vi "NI6602.Initialize.vi"(0 "i ref in":refnum<vi>, 2 "Counter Array":tag[](array[tag]), 5 "error in (no error)":errorcluster) -> (14 "i ref out":refnum<vi>, 16 "Task Array":refnum<k21>[](array[refnum]), 19 "error out":errorcluster)   [LabVIEW 2014, in "NI6602.lvlib"]
doc: "Initializes the device.\n\nLicense Agreement for this software:\n\nCopyright (C)\nGesellschaft für Schwerionenforschung, GSI\nPlanckstr. 1\n64291 Darmstadt\nGermany\n\nContact: D.Beck@gsi.de \n\nThis program is free software; you can redistribute it and/or modify it under the terms of the \nGNU General Public License as published by the Free Software Foundation; either version 2 of \nthe license, or (at your option) any later version.\n\nThis program is distributed in the hope that it will be useful, but WITHOUT ANY WARRANTY; \nwithout even the implied warranty of MERCHANTABILITY or FITNESS FOR A PARTICULAR PURPOSE. See the GNU General License for more details (http://www.gnu.org).\n\nGesellschaft für Schwerionenforschung, GSI\nPlanckstr. 1, 64291 Darmstadt, Germany\nFor all questions and ideas contact: M.Richter@gsi.de, H.Brand@gsi.de or D.Beck@gsi.de.\nLast update: 16-JUN-2004"
uses:
  NI6602.lvlib
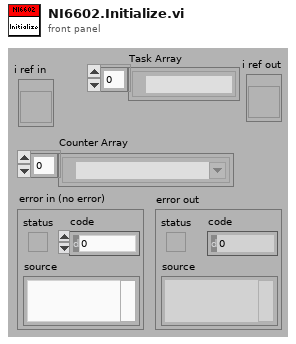
[diagram p1: front panel]
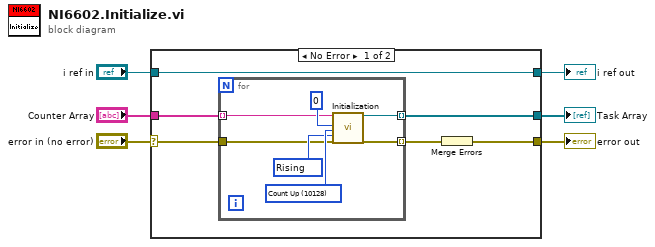
[diagram p0: block diagram]
diagram:
  n1 = case shown="No Error" "error in (no error)" {
    selector: "error in (no error)" -> [w9 w21]
    tunnel: [w10 w20] -> w6
    tunnel: [w11 w21] -> w5
    tunnel: "i ref in" -> [w10 w20]
    tunnel: "Counter Array" -> [w8 _]
    tunnel: [w7 _] -> w1
    frame No Error {
      n2 = for {
        tunnel: w9 -> [w16]
        tunnel: [w15] -> w12 mode=indexing
        tunnel: w8 -> [w14] mode=indexing
        tunnel: [w13] -> w7 mode=indexing
        w17 = 10280 items=["Rising"=10280, "Falling"=10171] ("edge")
        w18 = 10128 items=["Count Up"=10128, "Count Down"=10124, "Externally Controlled"=10326] ("count direction")
        n3 = call "Initialization.vi"("counter"=w14, "initial count"=u32 0, "count direction"=w18, "edge"=w17, "error in"=w16) -> ("task out"=w13:refnum<k21>, "error out"=w15:errorcluster)  [unwired: 13 in]
      }
      n4 = Merge Errors(w12) -> (w11:errorcluster)
    }
    frame Error {
    }
  }
  "i ref out" <- w6
  "error out" <- w5
  "Task Array" <- w1
